vi "ReadAvailableRecords.vi"(11 "scope params":T1={"scope mode"=enum."Stopped", "ticker"=refnum, "5160 samples per trigger"=0, "FPGA ref"=refnum, "P2P params"={"instrument handle"="", "stream session"=refnum, "scale"={"offset"=0.0, "gain"=0.0, "reserved 1"=0.0, "reserved 2"=0.0}, "actual sample rate"=10000000.0, "Trigger"=enum."PFI 0", "SCOPE Resource"="Dev1", "input impedance"=0}, "data mode"=enum."Real IO", "5782 samples per record"=0, "Chart length"=0} {"P2P params"."input impedance" items=["1 mega ohm"=0, "50 ohms"=2]; "P2P params"."actual sample rate" format="%.2p"}) -> (0 "last record size 5782":u32, 1 "last record size 5160":u32, 2 "record available":bool, 3 "scope params out":T1={"scope mode"=enum."Stopped", "ticker"=refnum, "5160 samples per trigger"=0, "FPGA ref"=refnum, "P2P params"={"instrument handle"="", "stream session"=refnum, "scale"={"offset"=0.0, "gain"=0.0, "reserved 1"=0.0, "reserved 2"=0.0}, "actual sample rate"=10000000.0, "Trigger"=enum."PFI 0", "SCOPE Resource"="Dev1", "input impedance"=0}, "data mode"=enum."Real IO", "5782 samples per record"=0, "Chart length"=0} {"P2P params"."input impedance" items=["1 mega ohm"=0, "50 ohms"=2]; "P2P params"."actual sample rate" format="%.2p"}, 4 "#elements 5160":u32, 6 "#elements 5782":u32)   [LabVIEW 2013]
uses:
  controls/scope_params.ctl
  Utilities/Ticker/Ticker.lvclass
  controls/ScopeMode.ctl
  Config/FPGAref.ctl
  P2P streaming/P2P params.ctl
  P2P streaming/trigger_source.ctl
  FPGA/DataMode.ctl
  <vilib>/rvi/interface/common/niFpgaWaitOnOcc.vi
  <vilib>/Utility/error.llb/Error Cluster From Error Code.vi
  <vilib>/rvi/errors/niLvFpgaAdjustHostInterfaceError.vi
  <vilib>/rvi/interface/nirviMethod/nirviMethod.xnode
  <vilib>/FPGAPlugInAG/Dynamic/niLvFpga_ReadFifo_Dynamic.vi
  <vilib>/rvi/errors/niLvFpgaMergeErrorWithErrorCode.vi
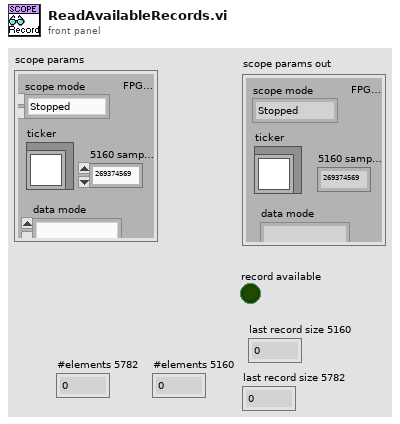
[diagram p1: front panel]
types:
  T1 = typedef "scope_params.ctl" = cluster{"scope mode":T2, "ticker":refnum<class "Ticker.lvclass">, "5160 samples per trigger":u32, "FPGA ref":T3, "P2P params":T4, "data mode":T6, "5782 samples per record":u32, "Chart length":i32}
  T2 = typedef "ScopeMode.ctl" = enum16{"Stopped", "Single", "Running", "Continuous"}
  T3 = typedef "FPGAref.ctl" = refnum<k20>
  T4 = typedef "P2P params.ctl" = cluster{"instrument handle":refnum<k15>, "stream session":refnum<k20>, "scale":cluster{"offset":dbl, "gain":dbl, "reserved 1":dbl, "reserved 2":dbl}, "actual sample rate":dbl, "Trigger":T5, "SCOPE Resource":refnum<k15>, "input impedance":u32}
  T5 = typedef "trigger_source.ctl" = enum16{"PFI 0", "PFI 1", "Software"}
  T6 = typedef "DataMode.ctl" = enum16{"Real IO", "Simulated"}
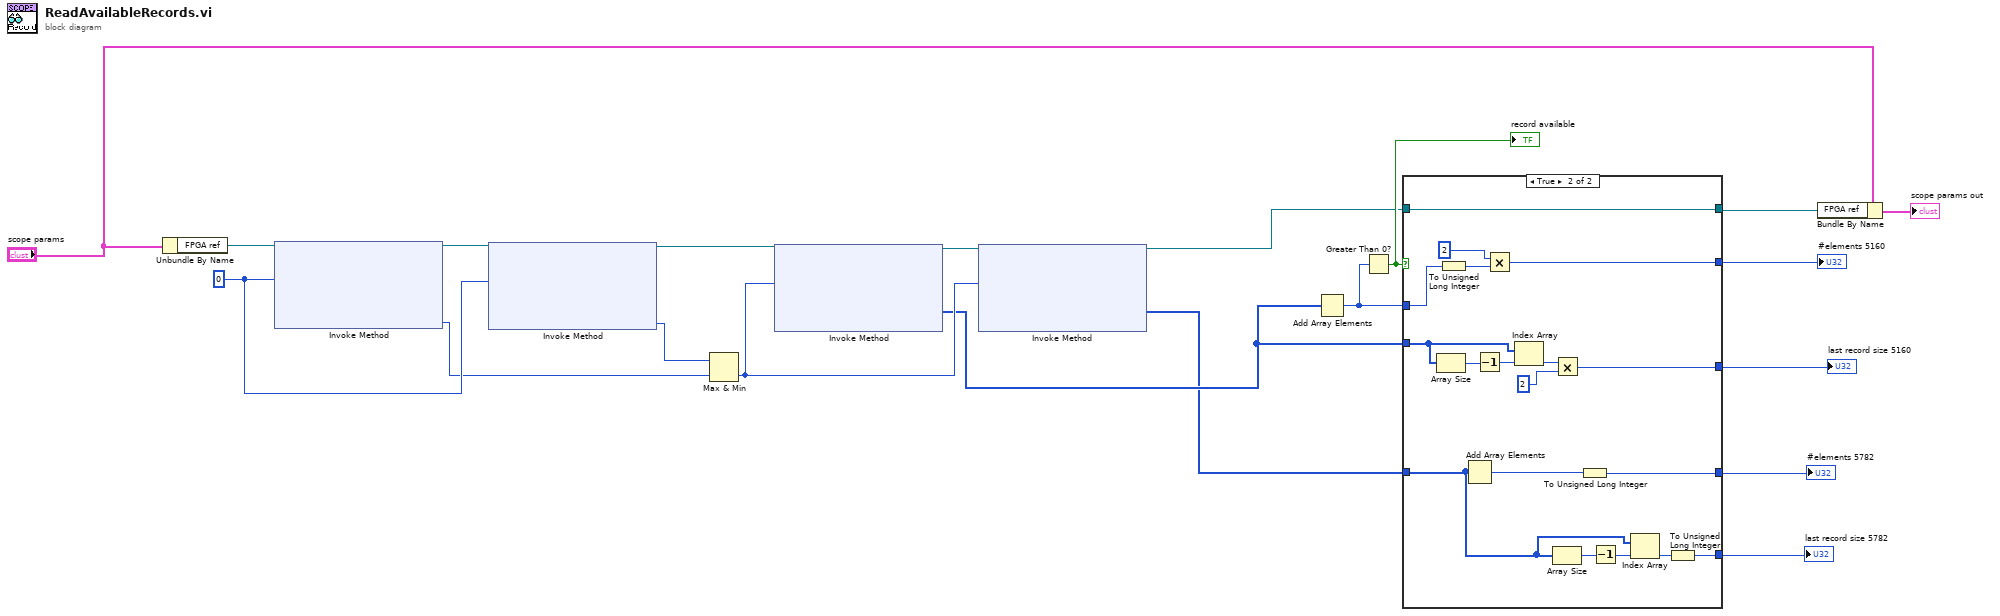
[diagram p0: block diagram]
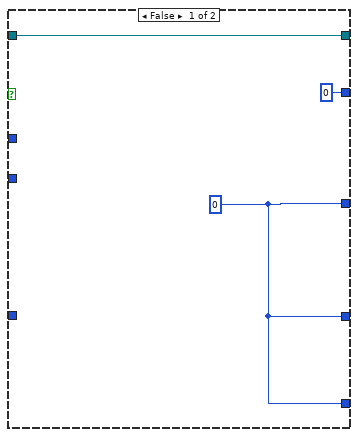
[diagram p2: hidden frame]
diagram:
  w12 = u32 0 ("Number of Elements")
  n1 = Unbundle By Name("scope params") -> ("FPGA ref"=w13:T3)
  n2 = xnode "Invoke Method"("FPGA VI Reference In"=w13, "Number of Elements"=w12) -> ("FPGA VI Reference Out"=w2:T3, "Elements Remaining"=w10:u32)  [unwired: 2 in, 2 out]
  n3 = xnode "Invoke Method"("FPGA VI Reference In"=w2, "Number of Elements"=w12) -> ("FPGA VI Reference Out"=w1:T3, "Elements Remaining"=w11:u32)  [unwired: 2 in, 2 out]
  n4 = Max & Min(x=w11, y=w10) -> (min(x,y)=w8:u32)  [unwired: 1 out]
  n5 = xnode "Invoke Method"("FPGA VI Reference In"=w1, "Number of Elements"=w8) -> ("FPGA VI Reference Out"=w9:T3, "Data"=w6:i32[])  [unwired: 2 in, 2 out]
  n6 = xnode "Invoke Method"("FPGA VI Reference In"=w9, "Number of Elements"=w8) -> ("FPGA VI Reference Out"=w7:T3, "Data"=w5:u16[])  [unwired: 2 in, 2 out]
  n7 = Add Array Elements(numeric array=w6) -> (sum=w20:i32)
  n8 = Greater Than 0?(x=w20) -> (x > 0?=w19:bool)
  "record available" <- w19
  n9 = case shown="True" w19 {
    tunnel: w7 -> [w23 w31]
    tunnel: w20 -> [_ w38]
    tunnel: w6 -> [_ w41]
    tunnel: [w23 w31] -> w14
    tunnel: [w21 w33] -> w16
    tunnel: [u32 0 w32] -> w15
    tunnel: w5 -> [_ w27]
    tunnel: [w21 w26] -> w4
    tunnel: [w21 w24] -> w3
    frame False {
      w21 = u32 0
    }
    frame True {
      n10 = Array Size(array=w41) -> (size(s)=w40:i32)
      n11 = To Unsigned Long Integer(number=w38) -> (unsigned 32bit integer=w37:u32)
      n12 = Add Array Elements(numeric array=w27) -> (sum=w30:u16)
      n13 = Decrement(x=w40) -> (x-1=w39:i32)
      n14 = Multiply(x=u32 2, y=w37) -> (x*y=w32:u32)
      n15 = Index Array(array=w41, index=w39) -> (element=w35:i32)
      n16 = Multiply(x=w35, y=u32 2 ("x")) -> (x*y=w33:u32)
      n17 = Array Size(array=w27) -> (size(s)=w29:i32)
      n18 = To Unsigned Long Integer(number=w30) -> (unsigned 32bit integer=w26:u32)
      n19 = Decrement(x=w29) -> (x-1=w28:i32)
      n20 = Index Array(array=w27, index=w28) -> (element=w25:u16)
      n21 = To Unsigned Long Integer(number=w25) -> (unsigned 32bit integer=w24:u32)
    }
  }
  "last record size 5160" <- w16
  "#elements 5160" <- w15
  "last record size 5782" <- w3
  "#elements 5782" <- w4
  n22 = Bundle By Name(cluster="scope params", "FPGA ref"=w14) -> (→"scope params out":T1)
